vi "Network-Order Bytes To Words Poly.vi"   [LabVIEW 2020, in "NI_Bit Manipulation.lvlib"]
doc: "Construct an array of integers from a byte array in network byte order, i.e. big-endian. This polymorphic VI wraps an underlying malleable VI."
uses:
  <vilib>/Bit Manipulation/NI_Bit Manipulation.lvlib
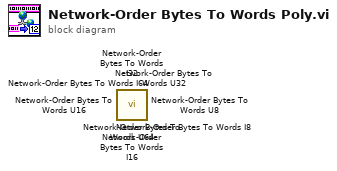
[diagram p0: block diagram]
diagram:
  n1 = call <vilib>:"Network-Order Bytes To Words U64.vi"() -> ()  [unwired: 1 in, 1 out]
  n2 = call <vilib>:"Network-Order Bytes To Words U32.vi"() -> ()  [unwired: 1 in, 1 out]
  n3 = call <vilib>:"Network-Order Bytes To Words U16.vi"() -> ()  [unwired: 1 in, 1 out]
  n4 = call <vilib>:"Network-Order Bytes To Words U8.vi"() -> ()  [unwired: 1 in, 1 out]
  n5 = call <vilib>:"Network-Order Bytes To Words I64.vi"() -> ()  [unwired: 1 in, 1 out]
  n6 = call <vilib>:"Network-Order Bytes To Words I32.vi"() -> ()  [unwired: 1 in, 1 out]
  n7 = call <vilib>:"Network-Order Bytes To Words I16.vi"() -> ()  [unwired: 1 in, 1 out]
  n8 = call <vilib>:"Network-Order Bytes To Words I8.vi"() -> ()  [unwired: 1 in, 1 out]
